vi "Find Child Attributes.vi"(7 "Actor in":refnum<class "Actor.lvclass">, 10 "Alias":string) -> (0 "Error out":errorcluster, 2 "Child Attributes":T1)   [LabVIEW 2020, in "jettl.lvlib" / "Actor Specific.lvlib"]
uses:
  Actor Specific.lvlib
  jettl.lvlib
  Actor/Actor.lvclass
  Unified Actor.ctl
  Msg/Msg.lvclass
  Msg Set.ctl
  Msg Input/Msg Input.lvclass
  Msg Output/Msg Output.lvclass
  Unified Actor Relation.ctl
  Teller.ctl
  Msg.ctl
  Msgs.ctl
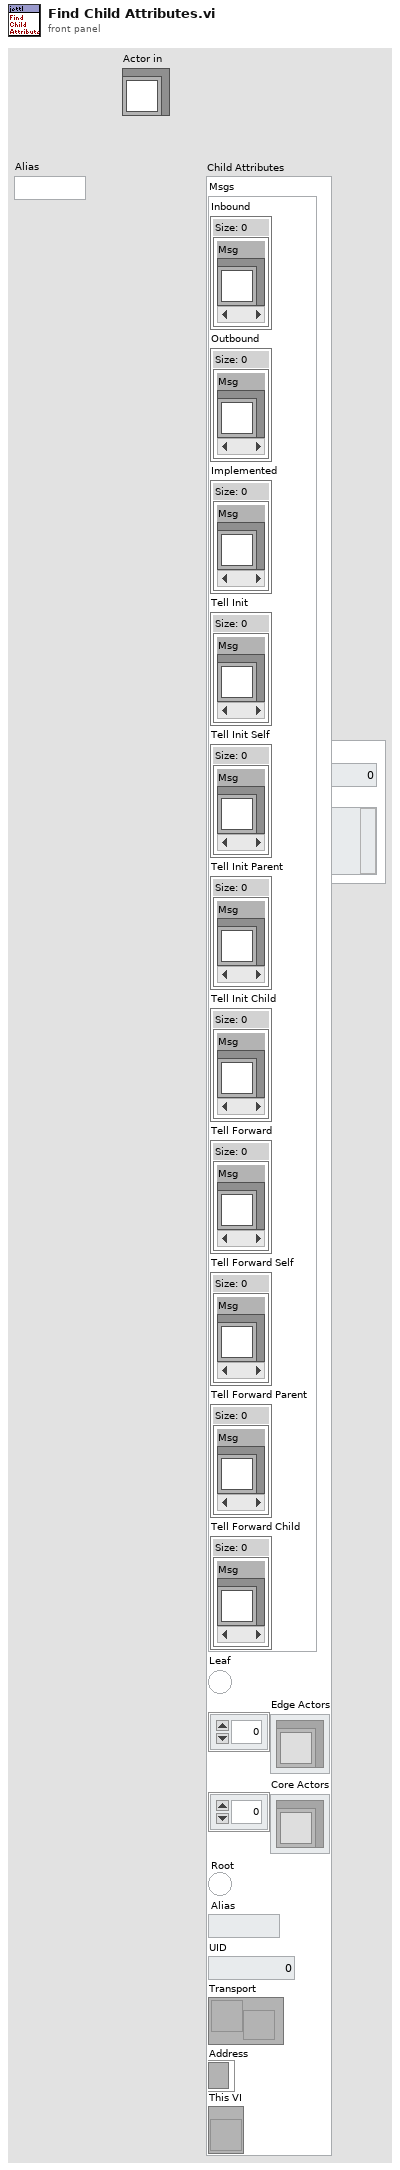
[diagram p1: front panel]
types:
  T1 = typedef "jettl.lvlib/Unified Actor.ctl" = cluster{"Msgs":T2, "Leaf":bool, "Edge Actors":refnum<class "Actor.lvclass">[], "Core Actors":refnum<class "Actor.lvclass">[], "Root":bool, "Alias":string, "UID":i32, "Transport":refnum<user-event>, "Address":refnum<event-registration>, "This VI":refnum<vi>}
  T2 = typedef "jettl.lvlib/Msgs.ctl" = cluster{"Inbound":T3, "Outbound":T3, "Implemented":T3, "Tell Init":T3, "Tell Init Self":T3, "Tell Init Parent":T3, "Tell Init Child":T3, "Tell Forward":T3, "Tell Forward Self":T3, "Tell Forward Parent":T3, "Tell Forward Child":T3}
  T3 = typedef "jettl.lvlib/Msg Set.ctl" = set{refnum<class "Msg.lvclass">}
  T4 = typedef "jettl.lvlib/Child Unified Actor.ctl" = map{string, T1}
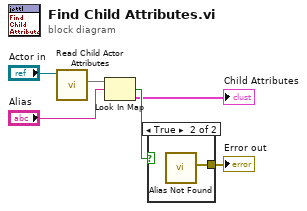
[diagram p0: block diagram]
diagram:
  n1 = call-dynamic "Read Child Actor Attributes.vi"("Actor in"="Actor in") -> ("Child Actor Attributes"=w2:T4)  [unwired: 10 in]
  n2 = Look In Map(map=w2, key="Alias") -> (key not found?=w5:bool, value=→"Child Attributes":T1)  [unwired: 1 in]
  n3 = case shown="True" w5 {
    tunnel: [_ w7] -> w4
    frame False {
    }
    frame True {
      n4 = call "Alias Not Found.vi"() -> ("Error"=w7:errorcluster)  [unwired: 11 in]
    }
  }
  "Error out" <- w4
